vi "Create Instance Impl.vi"(8 "error in (no error)":errorcluster, 10 "Configuration":T1, 11 "Newport Power Meter in":refnum<class "Newport Power Meter.lvclass">) -> (0 "error out":errorcluster, 3 "Newport Power Meter out":refnum<class "Newport Power Meter.lvclass">)   [LabVIEW 2023, in "Newport Power Meter.lvlib" / "Newport Power Meter.lvclass"]
uses:
  Newport Power Meter.lvclass
  Newport Power Meter.lvclass/Newport Power Meter.ctl
  <vilib>/Instr/_visa.llb/VISA Configure Serial Port (Instr).vi
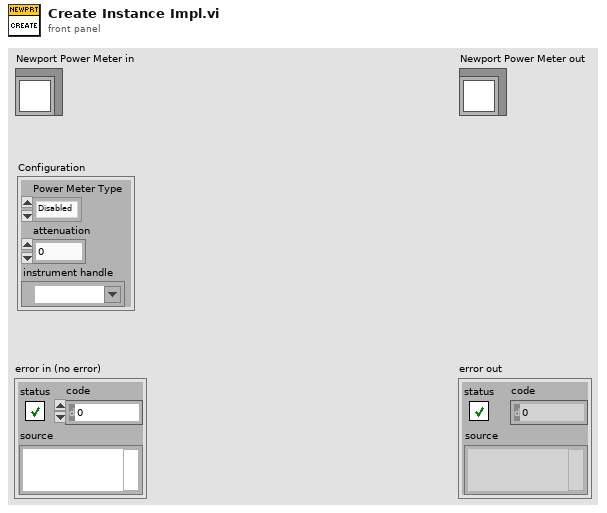
[diagram p1: front panel]
types:
  T1 = cluster{"Power Meter Type":enum16{"Disabled", "Thorlabs", "Newport", "Coherent"}, "attenuation":dbl, "instrument handle":refnum<visa-resource-name>}
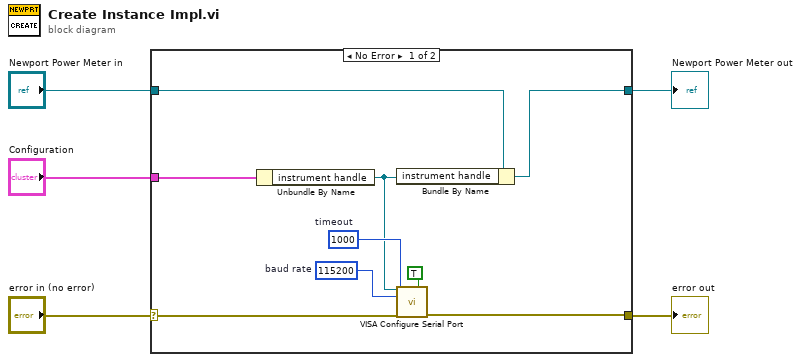
[diagram p0: block diagram]
diagram:
  n1 = case shown="No Error" "error in (no error)" {
    selector: "error in (no error)" -> [w8 w15]
    tunnel: "Configuration" -> [w14 _]
    tunnel: "Newport Power Meter in" -> [w13 w16]
    tunnel: [w12 w16] -> w2
    tunnel: [w7 w15] -> w1
    frame No Error {
      w10 = u32 1000  # timeout
      w6 = u32 115200  # baud rate
      n2 = Unbundle By Name(w14) -> ("instrument handle"=w9:refnum<visa-resource-name>)
      n3 = Bundle By Name(cluster=w13, "instrument handle"=w9) -> (w12:refnum<class "Newport Power Meter.lvclass">)
      n4 = call-poly "VISA Configure Serial Port"("VISA resource name"=w9, "timeout (10sec)"=w10, "Enable Termination\nChar (T)"=TRUE ("Enable Termination\nChar (T)"), "baud rate (9600)"=w6, "error in (no error)"=w8) -> ("error out"=w7:errorcluster)  [unwired: 9 in, 1 out]
    }
    frame Error {
    }
  }
  "error out" <- w1
  "Newport Power Meter out" <- w2
